vi "HFRR ADV v01.vi"() -> ()   [LabVIEW 2025] (continued)
  # "Choose which temperature sensor you are calibrating. Both use the same two-\npoint procedure: 0 °C (ice-point) and 60 °C (high-point)."
  # "Step 1 — Reference Instrument Setup"
  # "Connect a calibrated reference to the DUT port. This calibration performs two sets: one at 0 °C and one at 60 °C."
  # "Set A\n0 °C\nIce-point calibration"
  # "Set B\n60 °C\nHigh-point calibration"
  # "Allow the temperature bath to stabilise for at least 2 minutes at each set-point before recording the reading."
  # "Step 2 — Set A:  0 °C Calibration"
  # "Connect the  0 °C reference connector. Wait for the temperature to stabilise. Once stable, and click Record Point."
  # "Step 3 — Set B:  60 °C Calibration"
  # "Connect the  60 °C reference connector. Wait for the temperature to stabilise. Once stable, and click Record Point."
  # "Sample Temperature Calibration Complete"
  # "Sample Temperature Calibration PASSED\nMax deviation 0.200 °C — within ±0.5 °C tolerance. Two-point correction applied (0 °C & 60 °C)."
  # "Sample  Temperature Calibration Failed\nmeasured Sample Temperature differs from the factory calibration value"
  # "Step 1 — Reference Instrument Setup"
  # "Connect a calibrated reference to the DUT port. This calibration performs two sets: one at 0 °C and one at 60 °C."
  # "Set A\n0 °C\nIce-point calibration"
  # "Set B\n60 °C\nHigh-point calibration"
  # "Allow the temperature bath to stabilise for at least 2 minutes at each set-point before recording the reading."
  # "Step 2 — Set A:  0 °C Calibration"
  # "Connect the  0 °C reference connector. Wait for the temperature to stabilise. Once stable, and click Record Point."
  # "Step 3 — Set B:  60 °C Calibration"
  # "Connect the  60 °C reference connector. Wait for the temperature to stabilise. Once stable, and click Record Point."
  # "Air Temperature Calibration Complete"
  # "Air Temperature Calibration PASSED\nMax deviation 0.200 °C — within ±0.5 °C tolerance. Two-point correction applied (0 °C & 60 °C)."
  # "Air  Temperature Calibration Failed\nmeasured Sample Temperature differs from the factory calibration value"
  # "PID SAVE PARAMETERS"
  # "STROKE CALIBRATION"
  # "FF CALIBRATION"
  # "ABOUT SCREEN SAVE PARAMETERS"
  # "© 2023"
  # "System Control Commands\nS;1 - Starts the full automation cycle (Runs Priming-humidify till 70RH sequence first, then switches to Maintenance).\nS;0 - Stops the system immediately and enters Standby mode (Safe State: All actuators OFF).\nM;1 - Skips the priming sequence and jumps directly to Maintenance mode (PID control).\nR;1 - Resets the logic state machine and clears all errors, returning to Standby.\nService Mode (Manual Control)\nX;1 - Enters Manual Service Mode. This disables all automatic logic, sensor safety checks, and timers.\nX;0 - Exits Manual Service Mode and returns to Standby (Safe State).\nActuator Commands (Only work after sending X;1)\nP;[0-255] - Sets the Pump PWM. Note that this is Active Low (0 = Max Flow, 255 = Pump OFF).\nF;I;[0-255] - Sets the Intake Fan speed (0 = OFF, 255 = Max Speed).\nF;O;[0-255] - Sets the Exhaust Fan speed (0 = OFF, 255 = Max Speed).\nD;1 - Turns the Dehumidifier Relay ON.\nD;0 - Turns the Dehumidifier Relay OFF."
  # "%RH"
types:
  T1 = enum32{"Home", "Dashboard", "Imaging", "Report", "Analysis", "About", "Test Setup", "Advance", "Calibration"}
  T2 = typedef "imagedata.ctl" = cluster{"image type":i32, "image depth":i32, "image":u8[], "mask":u8[], "colors":u32[], "Rectangle":cluster{"left":i16, "top":i16, "right":i16, "bottom":i16}}
  T3 = enum32{"HOME", "Test Setup", "Acquire", "Compare Files", "Print Report", "About", "Advance", "Mooha"}
  T4 = enum32{"HOME", "Test Setup", "Acquire", "Adv Scar", "Adv Scar Report", "Compare Files", "Calibration", "About", "Advance", "Mooha"}
  T5 = enum16{"ASTM D6079", "ISO 12156", "CEC F-096-A-06", "Custom"}
  T6 = enum32{"Dashboard 1", "Dashboard 2", "Dashboard 3"}
  T7 = enum32{"COF", "Friction", "ECR", "Temperature", "Stroke"}
  T8 = enum32{"Coefficient Of Friction", "Air Temperature", "Humidity", "Stroke", "Sample Temperature", "Electrical Contact Resistance", "Frequency", "Air Temp vs Rh"}
  T9 = enum32{"Main", "Stroke", "Friction", "Temperature"}
  T10 = enum32{"Stroke Calibration", "Friction Force Calibration", "Temperature Calibration", "Default"}
  T11 = enum32{"Step 1", "Step 2", "Step 3", "Step 4", "Step 5", "Step 6", "Step 7", "Step 8", "Step 9"}
  T12 = enum32{"Test Progress", "Stroke Points Completed"}
  T13 = enum32{"Page 1", "Page 2", "Page 3", "Page 4", "Page 5", "Page 6"}
  T14 = enum32{"Main", "Step 1", "Step 2", "Step 3", "Step 4", "Air Step 1", "Air Step 2", "Air Step 3", "Air Step 4"}
  T15 = enum32{"Air Temperature", "Sample Temperature", "Default"}
  T16 = enum32{"COMMUNICATION", "CALIBRATION", "Temp Variables", "Camera", "WO 2472 (1)", "WO 2472 (2)", "WO 2472 (3)"}
  T17 = typedef "Auto Start enum.ctl" = enum16{"Init", "Humidity & Temperature On", "Reach point", "Maintain Stage", "Start Stage", "close", "Exit"}
  T18 = cluster{"Read Heave and Surge":string, "Bytes at Heave Port":dbl, "Heave and Surge COM Port:":refnum<visa-resource-name>, "Com Port 2":refnum<visa-resource-name>, "Residual Due":string, "Heave COM Status 2":bool, "Heave COM Status":bool, "Port 2":bool, "Sway PPR":dbl, "Surge PPR":dbl, "Heave PPR":dbl, "Sway Pitch":dbl, "Surge Pitch":dbl, "Heave Pitch":dbl, "Sway Pulses/mm":dbl, "Surge Pulses/mm":dbl, "Heave Pulses/mm":dbl, "inner loop":dbl, "Read Heave and Surge 2":string, "String 36":string, "Write S":bool, "WriteCC1":string[], "Heave COM Loop":i32, "LastCom":string, "EXIT":bool, "Error Heave":errorcluster}
  T19 = enum8{"Enabled", "Disabled", "Disabled and Grayed Out"}
  T20 = cluster{"Read Uno":string, "Bytes at Heave Port":dbl, "UNO COM Port:":refnum<visa-resource-name>, "UNO COM Port: 2":refnum<visa-resource-name>, "Residual Due":string, "UNO COM Status 2":bool, "UNO COM Status":bool, "Port 2":bool, "Sway PPR":dbl, "Surge PPR":dbl, "Heave PPR":dbl, "Sway Pitch":dbl, "Surge Pitch":dbl, "Heave Pitch":dbl, "Sway Pulses/mm":dbl, "Surge Pulses/mm":dbl, "Heave Pulses/mm":dbl, "inner loop":dbl, "Read Heave and Surge 2":string, "String 36":string, "Write S":bool, "WriteCC1":string[], "Heave COM Loop":i32, "LastCom":string, "EXIT":bool, "Error Heave":errorcluster}
  T21 = enum32{"HOME", "Test Setup", "Acquire", "Adv Scar", "Adv Scar Report", "Compare Files", "About", "Advance", "Mooha"}
  T22 = typedef "POST ANALYSIS ENUM.ctl" = enum16{"OPEN EXE", "INIT", "OPEN FILE", "FIT", "DRAW REC", "DRAW LINE", "PAN", "ZOOM IN", "ZOOM OUT", "SET ZOOM", "CLEAR ROI", "GET MEASUREMENTS", "RESIZE MODE", "STREAM START", "STREAM STOP", "SHOW UI", "MINIMIZE UI", "HIDE UI", "CKISE APP", "CLOSE CONNECTION", "SAVE IMAGE", "SET ROI COLOR", "READ", "TCP CHECK", "CLOSE"}
  T23 = typedef "CAMERA LIVE FEED ENUM.ctl" = enum16{"OPEN EXE", "INIT", "READ", "CAMERA CONNECT", "CAMERA START", "CAMERA STOP", "CAMERA GRAY", "CAMERA RGB", "CAMERA MINIMIZE", "CAMERA CLOSE", "CAMERA MODE LIST", "CAMERA MODE SET", "CAMERA RESTORE", "CAMERA SAVE", "CLOSE"}
  T24 = enum16{"Always On", "Always Off", "Off While Running"}
  T25 = enum32{"Home", "Dashboard", "Imaging", "Report", "Analysis", "About", "Test Setup", "Advance"}
  T26 = cluster{"File Name":string, "Test Method":string, "Operator":string, "Fuel Description":string, "Date and time":string}
  T27 = enum32{"Home", "Dashboard", "Imaging", "Report", "Analysis", "About", "Test Setup"}
  T28 = enum32{"HOME", "Test Setup", "Acquire", "Compare Files", "About", "Advance", "Mooha"}
  T29 = typedef "NI_ReportGenerationCore.lvlib/HTML Report Image Alignment.ctl" = enum16{"(default)", "LEFT", "RIGHT", "TOP", "TEXTTOP", "MIDDLE", "ABSMIDDLE", "BASELINE", "BOTTOM", "ABSBOTTOM"}
  T30 = cluster{"y":dbl, "LVDT STROKE DISPLAY":dbl, "y":dbl}
  T31 = enum16{"INIT", "READ", "MANUAL WRITE", "WRITE", "CLOSE", "ERROR INIT"}
diagram:
  w1 = FALSE
  w8 = 0.0 ("ch0_filt")
  w10 = -9999999.0 ("max_ch0")
  w11 = 9999999.0 ("min_ch0")
  w22 = FALSE ("Visible")
  w23 = T19."Enabled" ("Disabled")
  w26 = FALSE ("Visible")
  w25 = FALSE ("Humidity Off Command")
  w41 = "" ("USER ID")
  (unwired) T21."HOME" ("Main Tab")
  # "Temperature Continue Air Step 2"
  # "[CH1]    - FF\n[CH2]   - TEMPERATURE\n[CH3]    - Humidity\n[CH4]    - AIR TEMP\n[CH5]\\- Visa Uno\n[CH6] \\- Visa Due\n[CH7]  \\- file path\n[CH8]   - Displacement Gain\n[CHA]   - Stroke Gain\n[CHB]   - Stroke PID Gain\n[CHC]   -Language Selection\n[CHD]   -Power +\n[CHE]   -Power_\n[CHF]   -Heater\n[CHG]   -Humidity Wet\n[CHH]   -Humidity Dry\n[CHI]   -Integral Time \n[CHIJ   -Air intercept\n[CHI]   -Temp Intercept"
  n1 = local write "Cal Password"("" ("Cal Password")) -> ()
  n2 = property on="Auto Start Test" class="Bool (strict)"("Visible"=TRUE) -> ()  [unwired: 2 in, 2 out]
  n3 = property on="Friction Force Calibration Result Tab" class="TabCtl (strict)"("Visible"=FALSE) -> ()  [unwired: 2 in, 2 out]
  n4 = property on="FRICVALZ 2" class="Bool (strict)"("DisabledEnum"=w23) -> ()  [unwired: 2 in, 2 out]
  n5 = property on="FRICVALZ 4" class="Bool (strict)"("DisabledEnum"=w23) -> ()  [unwired: 2 in, 2 out]
  n6 = property on="FRICVALZ 3" class="Bool (strict)"("DisabledEnum"=w23) -> ()  [unwired: 2 in, 2 out]
  n7 = property on="About" class="Clust (strict)"("Visible"=FALSE) -> ()  [unwired: 2 in, 2 out]
  n8 = property on="Wrong Password" class="Str"("Visible"=w22) -> ()  [unwired: 2 in, 2 out]
  n9 = property on="Calibration 2" class="TabCtl (strict)"("Visible"=w22) -> ()  [unwired: 2 in, 2 out]
  n10 = local write "Temperature Selection"(T15."Default" ("Temperature Selection")) -> ()
  n11 = local write "Calibration Selection"(T10."Default" ("Calibration Selection")) -> ()
  n12 = flat-sequence {
    tunnel: [w77] -> w7
    tunnel: [w122] -> w33
    tunnel: w7 -> [w117]
    tunnel: [w123] -> w35
    tunnel: w33 -> [w123]
    tunnel: w35 -> [w183]
    tunnel: [w183] -> w34
    tunnel: w34 -> [w214]
    tunnel: [w214] -> w44
    tunnel: w44 -> [w221]
    tunnel: [w227] -> w32
    tunnel: [w215] -> w31
    tunnel: [w269] -> w6
    tunnel: [w268] -> _
    tunnel: w32 -> [w268]
    tunnel: w31 -> [w269]
    frame #0 {
      n13 = call "CLOSE CONNECTION.vi"("error in (no error)"="error in (no error) 2") -> ("error out"=w82:errorcluster)  [unwired: 10 in]
      n14 = call <vilib>:"Clear Errors.vi"("error in (no error)"=w82) -> ("error out"=w81:errorcluster)  [unwired: 5 in, 1 out]
      n15 = disable-structure shown="Enabled" {
        disable-tunnel: w81 -> [w109 _]
        disable-tunnel: [w108 _] -> w80
        frame Enabled {
          n16 = call <userlib>:"Fit VI window to Largest Dec.vi"("error in (no error)"=w109, "border spacing (2 px)"=1) -> ("error out"=w112:errorcluster, "dup VI Ref"=w116:refnum<vi>)  [unwired: 4 in]
          n17 = invoke on="Invoke Node" class="VI" method="FP.Run-Time Position.Maximized"(reference=w116, error in=w112) -> (error out=w113:errorcluster)  [unwired: 2 in, 3 out]
          n18 = call <vilib>:"Clear Errors.vi"("error in (no error)"=w113) -> ("error out"=w115:errorcluster)  [unwired: 5 in, 1 out]
          n19 = control-ref of="This VI"() -> (w107:refnum<vi>)
          n20 = invoke on="Invoke Node" class="VI" method="Default Vals.Reinit All"(reference=w107, error in=w115) -> (reference out=w111:refnum<vi>, error out=w110:errorcluster)  [unwired: 1 in, 1 out]
          n21 = Close Reference(reference=w111, error in (no error)=w110) -> (error out=w108:errorcluster)
        }
        frame Disabled {
        }
      }
      n22 = call "Stall Data Flow.vim"("value in"=w80, "milliseconds to wait"=u32 2000) -> ("value out"=w79:errorcluster)  [unwired: 1 out]
      n23 = call "Read Config.vi"("error in (no error)"=w79) -> ("error out"=w77:errorcluster, "STROKE PARAMETERS"=w88:dbl[], "ADC PARAMETERS"=w89:dbl[], "PID  PARAMETERS"=w90:dbl[], "CALIBRATION PARAMETERS"=w75:string[], "Stroke Calibration"=w87:string)  [unwired: 5 in]
      n24 = Index Array(array=w75) -> (element #1=w74:string, element #2=w73:string, element #3=w72:string, element #4=w71:string, element #5=w70:string, element #6=w68:string, element #7=w67:string, element #8=w66:string, element #9=w65:string, element #10=w64:string, element #11=w63:string, element #12=w62:string)  [unwired: 12 in]
      n25 = Index Array(array=w88) -> (element #1=w105:dbl, element #2=w106:dbl)  [unwired: 2 in]
      n26 = Index Array(array=w89) -> (element #1=w101:dbl, element #2=w102:dbl, element #3=w103:dbl, element #4=w104:dbl, element #5=w69:dbl)  [unwired: 5 in]
      n27 = Index Array(array=w90) -> (element #1=w92:dbl, element #2=w93:dbl, element #3=w94:dbl, element #4=w95:dbl, element #5=w96:dbl, element #6=w97:dbl, element #7=w98:dbl, element #8=w99:dbl, element #9=w100:dbl)  [unwired: 9 in]
      n28 = local write "STROKE FILTER"(w105) -> ()
      n29 = local write "Add up Stroke"(w106) -> ()
      n30 = local write "milliseconds to wait"(w92) -> ()
      n31 = local write "dt"(w93) -> ()
      n32 = local write "kp"(w94) -> ()
      n33 = local write "ki"(w95) -> ()
      n34 = local write "kd"(w96) -> ()
      n35 = local write "max_step_change"(w97) -> ()
      n36 = local write "max_amplitude"(w98) -> ()
      n37 = local write "min_amplitude"(w99) -> ()
      n38 = local write "startup_cmd"(w100) -> ()
      n39 = local write "VREF"(w101) -> ()
      n40 = local write "ADC_Resolution"(w102) -> ()
      n41 = local write "PIEZO_CAL_FACTOR"(w103) -> ()
      n42 = local write "NORMAL_FORCE"(w104) -> ()
      n43 = local write "Machine Serial Number"(w70) -> ()
      n44 = local write "STROKE CALIBRATION"(w74) -> ()
      n45 = local write "FRICTION CALIBRATION"(w73) -> ()
      n46 = local write "TEMPERATURE CALIBRATION"(w72) -> ()
      n47 = Fract/Exp String To Number(string=w71) -> (number=w76:dbl)  [unwired: 3 in, 1 out]
      n48 = local write "FF CAL EXCPTED VALUE"(w69) -> ()
      n49 = local write "version"(w68) -> ()
      n50 = local write "Version"(w67) -> ()
      n51 = local write "Workorder"(w66) -> ()
      n52 = local write "Runtime"(w65) -> ()
      n53 = local write "Firmware Version"(w64) -> ()
      n54 = local write "Operating System"(w63) -> ()
      n55 = local write "Instrument Serial"(w62) -> ()
      n56 = Spreadsheet String To Array(delimiter (Tab)=";", format string="", spreadsheet string=w87, array type (2D Dbl)=dbl[] []) -> (array=w91:dbl[])
      n57 = local write "Temperature diff"(w76) -> ()
      n58 = local write "calibration values"(w91) -> ()
    }
    frame #1 {
      n59 = property on="Auto Scar Check" class="Clust (strict)"("Visible"=TRUE) -> ()  [unwired: 2 in, 2 out]
      n60 = property on="Sign In" class="Bool (strict)"("DisabledEnum"=T19."Disabled" ("Disabled")) -> ()  [unwired: 2 in, 2 out]
      n61 = local write "sign in temp"(FALSE ("sign in temp")) -> ()
      n62 = call "dialog box.vi"("Status"="Before starting the test, verify that the microscope cable is connected.", "error in"=w117) -> ("error out"=w122:errorcluster)  [unwired: 8 in]
    }
    frame #2 {
      (unwired) TRUE ("Re-Initialise")
      # "kkkkk"
      # "C:\\Windows\\wndcm_pw_stdED hfrr.txt"
      # "C:\\LAB-IQ NXT"
      # "C:\\LAB-IQ NXT\\wndcm_pw_stdED hfrr.txt"
      # "password file"
      n63 = Current VI's Path() -> (path=w139:path)
      n64 = Strip Path(path=w139) -> (stripped path=w132:path)  [unwired: 1 out]
      n65 = local write "main tab sub"(enum32{"Page 1", "Page 2"}."Page 1" ("main tab sub")) -> ()
      n66 = local write "Main Tab Display"(T6."Dashboard 1" ("Main Tab Display")) -> ()
      n67 = local write "Main Tab"(T4."HOME" ("Main Tab")) -> ()
      n68 = Path To String(path=w132) -> (string=w134:string)
      n69 = Search/Split String(string=w134, search string/char (-)=".exe") -> (match + rest of string=w136:string)  [unwired: 1 in, 2 out]
      n70 = Match True/False String(2:".vi" ("false string"), 3:".exe" ("true string"), 4:w136) -> (0:w133:bool)  [unwired: 1 out]
      n71 = List Folder(path=path "C:/LAB-IQ" ("directory path"), pattern="*.txt") -> (filenames=w145:string[])  [unwired: 2 in, 3 out]
      n72 = case shown="True" w133 {
        tunnel: w132 -> [w154 w156]
        tunnel: [w154 w155] -> w130
        frame False {
        }
        frame True {
          n73 = Strip Path(path=w156) -> (stripped path=w155:path)  [unwired: 1 out]
        }
      }
      n74 = Search 1D Array(1D array=w145, element="wndcm_pw_stdED hfrr.txt") -> (index of element=w148:i32)  [unwired: 1 in]
      n75 = Equal?(x=w148, y=-1) -> (x = y?=w143:bool)
      n76 = Path To String(path=w130) -> (string=→"Gain path":string)
      n77 = case shown="True" w143 {
        frame False {
        }
        frame True {
          n78 = String To Byte Array(string="123\n") -> (unsigned byte array=w161:u8[])
          n79 = Array Size(array=w161) -> (size(s)=w160:i32)
          n80 = for {
            N: w160 -> [_]
            tunnel: w161 -> [w174]
            tunnel: [w171] -> w163 mode=indexing
            tunnel: w160 -> [w166]
            i -> [w164]
            n81 = Decrement(x=w166) -> (x-1=w167:i32)
            n82 = Index Array(array=w174, index=w164) -> (element=w173:u8)
            n83 = Equal?(x=w164, y=w167) -> (x = y?=w168:bool)
            n84 = Number To Decimal String(number=w173) -> (decimal integer string=w172:string)  [unwired: 1 in]
            n85 = Select(t="", s=w168, f="\r") -> (s? t:f=w165:string)
            n86 = Concatenate Strings(w172, w165) -> (w171:string)
          }
          n87 = local read "file path"() -> (w157:path)
          n88 = Concatenate Strings(w163) -> (w159:string)
          n89 = call <vilib>:"Write Characters To File.vi"("append to file? (new file:F)"=FALSE, "character string"=w159, "file path (dialog if empty)"=w157) -> ()  [unwired: 2 in, 1 out]
        }
      }
      n90 = local write "conststatus"(0.0 ("rpm value : 2")) -> ()
      n91 = local write "EVENT LOG"("") -> ()
      n92 = local write "COUNT"(0 ("COUNT")) -> ()
      n93 = local write "clk"(0.0 ("clk")) -> ()
      n94 = local write "Flag"(0.0 ("Flag")) -> ()
      n95 = local write "Lan flag"(0.0 ("Lan flag")) -> ()
      n96 = local write "Com flag"(u32 0 ("Com flag")) -> ()
      n97 = local write "refresh flag"(FALSE ("refresh flag")) -> ()
      "file path" <- path "C:/LAB-IQ/wndcm_pw_stdED hfrr.txt" ("file path")
      "FF buffer" <- dbl[] [] ("FF buffer")
    }
    frame #3 {
      # "C:\\WinDucom\\calibrate WO 2391.dcf"
      n98 = String To Path(string="C:\\LAB-IQ\\Image Calibrate v01.dcf") -> (path=w178:path)
      n99 = String To Path(string="C:\\LAB-IQ\\calibrate WO 2472.dcf") -> (path=w182:path)
      n100 = Open/Create/Replace File "Open File"(file path (use dialog)=w182) -> (refnum out=w181:refnum<file>)  [unwired: 5 in, 2 out]
      n101 = Open/Create/Replace File ("Open File")(file path (use dialog)=w178) -> (refnum out=w177:refnum<file>)  [unwired: 5 in, 2 out]
      n102 = for {
        N: 4 -> [_]
        tunnel: w177 -> [w189]
        i -> [w185]
        n103 = Read from Text File ("Read File")(file (use dialog)=w189) -> (text=w190:string)  [unwired: 3 in, 3 out]
        n104 = String Subset(string=w190, offset (0)=6, length (rest)=10 ("length (rest)")) -> (substring=w186:string)
        n105 = Fract/Exp String To Number(string=w186) -> (number=w184:dbl)  [unwired: 3 in, 1 out]
        n106 = case shown="3" w185 {
          tunnel: w184 -> [w191 w192 _ w193 _]
          frame 0 {
            n107 = local write "5x Gain"(w191) -> ()
          }
          frame 1 {
            n108 = local write "10x Gain"(w192) -> ()
          }
          frame 2 {
          }
          frame 3 {
            n109 = local write "100x gain"(w193) -> ()
          }
          frame 4, Default {
          }
        }
      }
      n110 = for {
        N: 24 -> [_]
        tunnel: w181 -> [w202]
        i -> [w196]
        (unwired) TRUE ("line mode (F)")
        n111 = Read from Text File "Read File"(file (use dialog)=w202) -> (text=w201:string)  [unwired: 3 in, 3 out]
        n112 = Match Pattern(string=w201, regular expression="]") -> (after substring=w199:string)  [unwired: 1 in, 3 out]
        n113 = String Subset(string=w201, offset (0)=5, length (rest)=10 ("length (rest)")) -> (substring=w194:string)
        n114 = Fract/Exp String To Number(string=w194) -> (number=w195:dbl)  [unwired: 3 in, 1 out]
        n115 = Match Pattern(string=w199, regular expression="-") -> (before substring=w197:string)  [unwired: 1 in, 3 out]
        n116 = case shown="18" w196 {
          tunnel: w195 -> [_ _ _ _ _ _ _ _ _ _ w209 _ _ _ _ _ _ _ _ _ _ _ _ _ _]
          tunnel: w197 -> [_ _ _ _ w205 w206 w207 _ _ _ _ _ _ _ _ _ _ _ _ _ w210 _ w211 w212 _]
          frame 0 {
          }
          frame 1 {
          }
          frame 2 {
          }
          frame 3 {
          }
          frame 4 {
            n117 = local write "Com Port 1"(w205) -> ()
          }
          frame 5 {
            n118 = local write "Com Port 2"(w206) -> ()
            n119 = local write "visa due"(w206) -> ()
          }
          frame 6 {
            n120 = String To Path(string=w207) -> (path=w208:path)
            n121 = local write "File Path"(w208) -> ()
          }
          frame 7 {
          }
          frame 8 {
          }
          frame 9 {
          }
          frame 10 {
            n122 = local write "Language Selection"(w209) -> ()
          }
          frame 11 {
          }
          frame 12 {
          }
          frame 13 {
          }
          frame 14 {
          }
          frame 15 {
          }
          frame 16 {
          }
          frame 17 {
          }
          frame 18 {
          }
          frame 21 {
          }
          frame 22 {
            n123 = local write "Com Port 3"(w210) -> ()
          }
          frame 23 {
          }
          frame 19 {
            n124 = local write "C3 :"(w211) -> ()
          }
          frame 20 {
            n125 = local write "Camera Port :"(w212) -> ()
          }
          frame 24, Default {
          }
        }
      }
    }
    frame #4 {
      n126 = Wait (ms)(milliseconds to wait=u32 1000) -> ()  [unwired: 1 out]
    }
    frame #5 {
      w230 = u32 2000 ("milliseconds to wait")
      w257 = u32 2000 ("milliseconds to wait")
      n127 = call "CAMERA LIVE FEED FGV.vi"("Enum - Menu"=CAMERA_LIVE_FEED_ENUM."OPEN EXE", "error in (no error)"=w221) -> ("error out"=w263:errorcluster)  [unwired: 8 in, 1 out]
      n128 = call "IMAGE ANALYSIS.vi"("Enum"=POST_ANALYSIS_ENUM."OPEN EXE", "error in"=w221) -> ("error out"=w218:errorcluster)  [unwired: 8 in, 1 out]
      n129 = call "Stall Data Flow.vim"("value in"=w263, "milliseconds to wait"=w257) -> ("value out"=w261:errorcluster)  [unwired: 1 out]
      n130 = call "Stall Data Flow.vim"("value in"=w218, "milliseconds to wait"=u32 8000) -> ("value out"=w217:errorcluster)  [unwired: 1 out]
      n131 = call "CAMERA LIVE FEED FGV.vi"("Enum - Menu"=CAMERA_LIVE_FEED_ENUM."INIT", "error in (no error)"=w261) -> ("error out"=w259:errorcluster)  [unwired: 8 in, 1 out]
      n132 = call "IMAGE ANALYSIS.vi"("Enum"=POST_ANALYSIS_ENUM."INIT", "error in"=w217) -> ("error out"=w215:errorcluster)  [unwired: 8 in, 1 out]
      n133 = case shown="Error .." w259 {
        selector: w259 -> [w264 _]
        tunnel: [w264 _] -> w258
        frame No Error {
        }
        frame Error {
          n134 = One Button Dialog(message="Camera initialization error.\nPlease Restart the software") -> ()  [unwired: 1 in, 1 out]
        }
      }
      n135 = property on="Camera Port :" class="CmbBox"() -> ("Strings[]"=w255:string[], "Value"=w256:string)  [unwired: 2 in, 2 out]
      n136 = Search 1D Array(1D array=w255, element=w256) -> (index of element=w254:i32)  [unwired: 1 in]
      n137 = Type Cast(type=30, x=w254) -> (*(type *) &x=w252:i32)
      n138 = call "Stall Data Flow.vim"("value in"=w258, "milliseconds to wait"=w257) -> ("value out"=w234:errorcluster)  [unwired: 1 out]
      n139 = Add(x=w252, y=48) -> (x+y=w233:i32)
      n140 = call "CAMERA LIVE FEED FGV.vi"("Enum - Menu"=CAMERA_LIVE_FEED_ENUM."CAMERA CONNECT", "error in (no error)"=w234, "CAMERA PORT"=w233) -> ("error out"=w243:errorcluster)  [unwired: 7 in, 1 out]
      n141 = call "Stall Data Flow.vim"("value in"=w243, "milliseconds to wait"=u32 5000) -> ("value out"=w244:errorcluster)  [unwired: 1 out]
      n142 = call "CAMERA LIVE FEED FGV.vi"("Enum - Menu"=CAMERA_LIVE_FEED_ENUM."CAMERA MODE LIST", "error in (no error)"=w244) -> ("error out"=w246:errorcluster)  [unwired: 8 in, 1 out]
      n143 = call "Stall Data Flow.vim"("value in"=w246, "milliseconds to wait"=w230) -> ("value out"=w245:errorcluster)  [unwired: 1 out]
      n144 = call "CAMERA LIVE FEED FGV.vi"("Enum - Menu"=CAMERA_LIVE_FEED_ENUM."READ", "error in (no error)"=w245) -> ("error out"=w232:errorcluster, "data out"=→"Camera List":string)  [unwired: 8 in]
      n145 = Type Cast(type=30, x=0) -> (*(type *) &x=w226:i32)
      n146 = call "Stall Data Flow.vim"("value in"=w232, "milliseconds to wait"=w230) -> ("value out"=w231:errorcluster)  [unwired: 1 out]
      n147 = Add(x=w226, y=48) -> (x+y=w224:i32)
      n148 = call "CAMERA LIVE FEED FGV.vi"("Enum - Menu"=CAMERA_LIVE_FEED_ENUM."CAMERA MODE SET", "error in (no error)"=w231, "CAMERA MODE"=w224) -> ("error out"=w228:errorcluster)  [unwired: 7 in, 1 out]
      n149 = call "Stall Data Flow.vim"("value in"=w228, "milliseconds to wait"=u32 2000) -> ("value out"=w248:errorcluster)  [unwired: 1 out]
      n150 = call "CAMERA LIVE FEED FGV.vi"("Enum - Menu"=CAMERA_LIVE_FEED_ENUM."CAMERA START", "error in (no error)"=w248) -> ("error out"=w249:errorcluster)  [unwired: 8 in, 1 out]
      n151 = call "Stall Data Flow.vim"("value in"=w249, "milliseconds to wait"=u32 1000) -> ("value out"=w250:errorcluster)  [unwired: 1 out]
      n152 = call "CAMERA LIVE FEED FGV.vi"("Enum - Menu"=CAMERA_LIVE_FEED_ENUM."CAMERA MINIMIZE", "error in (no error)"=w250) -> ("error out"=w227:errorcluster)  [unwired: 8 in, 1 out]
    }
    frame #6 {
      n153 = case shown="No Error" w268 {
        frame No Error {
          n154 = property on="Auto Scar Check" class="Clust (strict)"("Visible"=FALSE) -> ()  [unwired: 2 in, 2 out]
        }
        frame Error {
        }
      }
      n155 = property on="Sign In" class="Bool (strict)"("DisabledEnum"=T19."Enabled" ("Disabled")) -> ()  [unwired: 2 in, 2 out]
      n156 = local write "sign in temp"(TRUE ("sign in temp")) -> ()
    }
  }
  n157 = local write "SCAR MEASURMENT"(enum32{"Auto Scar", "Manual Scar"}."Manual Scar" ("SCAR MEASURMENT")) -> ()
  n158 = property on="Service Left" class="Bool (strict)"("Visible"=w1) -> ()  [unwired: 2 in, 2 out]
  n159 = property on="Service Right" class="Bool (strict)"("Visible"=w1) -> ()  [unwired: 2 in, 2 out]
  n160 = property on="Service Bottom" class="Bool (strict)"("Visible"=w1) -> ()  [unwired: 2 in, 2 out]
  n161 = local write "Temperature Off Command"(w25) -> ()
  n162 = local write "Main Dashboard Buttons"(T1."Home" ("Main Dashboard Buttons")) -> ()
  n163 = property on="Tab Control 6" class="TabCtl (strict)"("Visible"=FALSE) -> ()  [unwired: 2 in, 2 out]
  n164 = local write "Humidity Off Command"(w25) -> ()
  n165 = local write "CAMERA ROI MIN TEMP"(w25) -> ()
  n166 = local write "TEST FILE NAM,E SAVED"(w25) -> ()
  n167 = local write "LIVE FEED MIN TEMP"(w25) -> ()
  n168 = local write "SCAR MEASURMENT"(enum32{"Auto Scar", "Manual Scar"}."Manual Scar" ("SCAR MEASURMENT")) -> ()
  n169 = local write "Auto stop temp"(w26) -> ()
  n170 = local write "main tab sub"(enum32{"Page 1", "Page 2"}."Page 1" ("main tab sub")) -> ()
  n171 = while {
    stop <- w283 stop-if-true
    n172 = local read "Ambient Temperature"() -> (w281:dbl)
    n173 = Wait (ms)(milliseconds to wait=u32 200) -> ()  [unwired: 1 out]
    n174 = local read "Sample Temperature 2"() -> (w280:dbl)
    n175 = local write "Sensor value"(w281) -> ()
    n176 = local write "Sensor value"(w281) -> ()
    n177 = local write "Sensor value"(w280) -> ()
    n178 = local write "Sensor value"(w280) -> ()
    n179 = local write "Temperature — Live (Set A: 0 °C)"(w281) -> ()
    n180 = local write "Temperature — Live (Set A: 60 °C)"(w281) -> ()
    n181 = local write "Temperature — Live (Set A: 60 °C)"(w280) -> ()
    n182 = local write "Temperature — Live (Set A: 0 °C)"(w280) -> ()
    n183 = case shown="True" "Save Button" {
      selector: "Save Button" -> [_ w353]
      frame False {
      }
      frame True {
        n184 = Not(x=w353) -> (.not. x?=w352:bool)
        n185 = local read "Temperature diff"() -> (w349:dbl)
        n186 = local read "Machine Serial Number"() -> (w338:string)
        n187 = local read "milliseconds to wait"() -> (w385:u32)
        n188 = local write "Save Button"(w352) -> ()
        n189 = local read "max_step_change"() -> (w390:dbl)
        n190 = local read "FF CAL EXCPTED VALUE"() -> (w336:dbl)
        n191 = local read "Operating System"() -> (w329:string)
        n192 = local read "Firmware Version"() -> (w330:string)
        n193 = local read "max_amplitude"() -> (w391:dbl)
        n194 = local read "min_amplitude"() -> (w392:dbl)
        n195 = local read "Instrument Serial"() -> (w328:string)
        n196 = local read "PIEZO_CAL_FACTOR"() -> (w396:dbl)
        n197 = local read "startup_cmd"() -> (w393:dbl)
        n198 = local read "NORMAL_FORCE"() -> (w397:dbl)
        n199 = local read "ADC_Resolution"() -> (w395:dbl)
        n200 = local read "Workorder"() -> (w332:string)
        n201 = local read "Runtime"() -> (w331:string)
        n202 = local read "Version"() -> (w333:string)
        n203 = local read "version"() -> (w334:string)
        n204 = local read "kp"() -> (w387:dbl)
        n205 = local read "kd"() -> (w389:dbl)
        n206 = local read "calibration values"() -> (w400:dbl[])
        n207 = local read "dt"() -> (w386:dbl)
        n208 = local read "ki"() -> (w388:dbl)
        n209 = local read "STROKE FILTER"() -> (w398:i32)
        n210 = local read "Add up Stroke"() -> (w399:dbl)
        n211 = Number To Fractional String(number=w349) -> (F-format string=w348:string)  [unwired: 3 in]
        n212 = local read "VREF"() -> (w394:dbl)
        n213 = Insert Into Array(array=dbl[] [], new element #1=w385, new element #2=w386, new element #3=w387, new element #4=w388, new element #5=w389, new element #6=w390, new element #7=w391, new element #8=w392, new element #9=w393) -> (w401:dbl[])  [unwired: 1 in]
        n214 = Insert Into Array(array=dbl[] [], new element #1=w394, new element #2=w395, new element #3=w396, new element #4=w397, new element #5=w336) -> (w402:dbl[])  [unwired: 1 in]
        n215 = Array To Spreadsheet String(delimiter (Tab)=";", array=w400, 3:"" ("format string")) -> (spreadsheet string=w404:string)
        n216 = Insert Into Array(array=dbl[] [], new element #1=w398, new element #2=w399) -> (w403:dbl[])  [unwired: 1 in]
        n217 = Insert Into Array(array=string[] [], new element #1="STROKE CALIBRATION", new element #2="FRICTION CALIBRATION", new element #3="TEMPERATURE CALIBRATION", new element #4=w348, new element #5=w338, new element #6=w334, new element #7=w333, new element #8=w332, new element #9=w331, new element #10=w330, new element #11=w329, new element #12=w328) -> (w350:string[])  [unwired: 1 in]
        n218 = call "Write Config.vi"("Stroke Calibration"=w404, "CALIBRATION PARAMETERS"=w350, "STROKE PARAMETERS"=w403, "ADC PARAMETERS"=w402, "PID  PARAMETERS"=w401) -> ("error out"=w383:errorcluster)  [unwired: 6 in]
        n219 = call "Stall Data Flow.vim"("value in"=w383, "milliseconds to wait"=u32 2000) -> ("value out"=w384:errorcluster)  [unwired: 1 out]
        n220 = call "Read Config.vi"("error in (no error)"=w384) -> ("STROKE PARAMETERS"=w381:dbl[], "ADC PARAMETERS"=w380:dbl[], "PID  PARAMETERS"=w379:dbl[], "CALIBRATION PARAMETERS"=w344:string[], "Stroke Calibration"=w382:string)  [unwired: 5 in, 1 out]
        n221 = Index Array(array=w344) -> (element #1=w341:string, element #2=w340:string, element #3=w339:string, element #4=w343:string, element #5=w337:string, element #6=w327:string, element #7=w326:string, element #8=w325:string, element #9=w324:string, element #10=w323:string, element #11=w322:string, element #12=w321:string)  [unwired: 12 in]
        n222 = Index Array(array=w379) -> (element #1=w377:dbl, element #2=w376:dbl, element #3=w375:dbl, element #4=w374:dbl, element #5=w373:dbl, element #6=w372:dbl, element #7=w371:dbl, element #8=w370:dbl, element #9=w369:dbl)  [unwired: 9 in]
        n223 = Index Array(array=w380) -> (element #1=w368:dbl, element #2=w367:dbl, element #3=w366:dbl, element #4=w365:dbl, element #5=w335:dbl)  [unwired: 5 in]
        n224 = Index Array(array=w381) -> (element #1=w364:dbl, element #2=w363:dbl)  [unwired: 3 in, 1 out]
        n225 = Spreadsheet String To Array(delimiter (Tab)=";", format string="", spreadsheet string=w382, array type (2D Dbl)=dbl[] []) -> (array=w378:dbl[])
        n226 = local write "STROKE FILTER"(w364) -> ()
        n227 = local write "Add up Stroke"(w363) -> ()
        n228 = local write "VREF"(w368) -> ()
        n229 = local write "ADC_Resolution"(w367) -> ()
        n230 = local write "PIEZO_CAL_FACTOR"(w366) -> ()
        n231 = local write "NORMAL_FORCE"(w365) -> ()
        n232 = local write "FF CAL EXCPTED VALUE"(w335) -> ()
        n233 = local write "STROKE CALIBRATION"(w341) -> ()
        n234 = local write "FRICTION CALIBRATION"(w340) -> ()
        n235 = local write "TEMPERATURE CALIBRATION"(w339) -> ()
        n236 = Fract/Exp String To Number(string=w343) -> (number=w342:dbl)  [unwired: 3 in, 1 out]
        n237 = local write "Machine Serial Number"(w337) -> ()
        n238 = local write "version"(w327) -> ()
        n239 = local write "Version"(w326) -> ()
        n240 = local write "Workorder"(w325) -> ()
        n241 = local write "Runtime"(w324) -> ()
        n242 = local write "Firmware Version"(w323) -> ()
        n243 = local write "Operating System"(w322) -> ()
        n244 = local write "Instrument Serial"(w321) -> ()
        n245 = local write "calibration values"(w378) -> ()
        n246 = local write "milliseconds to wait"(w377) -> ()
        n247 = local write "dt"(w376) -> ()
        n248 = local write "kp"(w375) -> ()
        n249 = local write "ki"(w374) -> ()
        n250 = local write "kd"(w373) -> ()
        n251 = local write "max_step_change"(w372) -> ()
        n252 = local write "max_amplitude"(w371) -> ()
        n253 = local write "min_amplitude"(w370) -> ()
        n254 = local write "startup_cmd"(w369) -> ()
        n255 = local write "Temperature diff"(w342) -> ()
      }
    }
    n256 = local read "USER ID"() -> (w278:string)
    n257 = local read "run test Calibration"() -> (w276:bool)
    n258 = disable-structure shown="Enabled" {
      disable-tunnel: [w290 w301] -> w277
      frame Disabled {
        n259 = local read "Point 1 - 0.2 mm"() -> (w300:bool)
        n260 = local read "Point 2 - 0.4 mm"() -> (w299:bool)
        n261 = local read "Point 3 - 0.6 mm"() -> (w298:bool)
        n262 = local read "Point 4 - 0.8 mm"() -> (w297:bool)
        n263 = local read "Point 5 - 1.0 mm"() -> (w296:bool)
        n264 = local read "Point 6 - 1.2 mm"() -> (w295:bool)
        n265 = And(x=w300, y=w299) -> (x .and. y?=w294:bool)
        n266 = And(x=w298, y=w297) -> (x .and. y?=w293:bool)
        n267 = And(x=w296, y=w295) -> (x .and. y?=w291:bool)
        n268 = And(x=w294, y=w293) -> (x .and. y?=w292:bool)
        n269 = And(x=w292, y=w291) -> (x .and. y?=w290:bool)
      }
      frame Enabled {
        n270 = local read "Point 5 - 1.0 mm"() -> (w301:bool)
      }
    }
    n271 = local read "START TEMP"() -> (w275:bool)
    n272 = local write "tested by 2"(w278) -> ()
    n273 = And(x=w275, y=w276) -> (x .and. y?=w274:bool)
    n274 = case shown="True" w274 {
      frame False {
        w302 = TRUE ("PAUSE")
        n275 = call "ELAPSED TIMER VI - Calibration.vi"("RESET"=w302, "PAUSE"=w302) -> ()  [unwired: 7 in, 3 out]
      }
      frame True {
        w305 = FALSE ("PAUSE")
        n276 = call "ELAPSED TIMER VI - Calibration.vi"("TARGET"=60.0, "RESET"=w305, "PAUSE"=w305) -> ("ELAPSED INDICATION"=w303:bool)  [unwired: 6 in, 2 out]
        n277 = case shown="False" w303 {
          frame False {
            n278 = local write "Friction Force Calibration Result Tab"(enum32{"Calibration Results", "Page 2"}."Calibration Results" ("Friction Force Calibration Result Tab")) -> ()
            n279 = property on="Friction Force Calibration Result Tab" class="TabCtl (strict)"("Visible"=FALSE) -> ()  [unwired: 2 in, 2 out]
          }
          frame True {
            n280 = stacked-sequence {
              frame #0 {
                n281 = local read "Friction"() -> (→"Friction cal":dbl)
                n282 = local write "run test Calibration"(FALSE ("run test Calibration")) -> ()
                n283 = local write "START TEMP"(FALSE ("START TEMP")) -> ()
              }
              frame #1 {
                n284 = Wait (ms)(milliseconds to wait=u32 1500) -> ()  [unwired: 1 out]
              }
              frame #2 {
                n285 = local write "Due Write"("VC;0") -> ()
              }
              frame #3 {
                n286 = Wait (ms)(milliseconds to wait=u32 1500) -> ()  [unwired: 1 out]
              }
              frame #4 {
                n287 = local write "Due Write"("VC;0") -> ()
              }
              frame #5 {
                n288 = property on="Friction Force Calibration Result Tab" class="TabCtl (strict)"("Visible"=TRUE) -> ()  [unwired: 2 in, 2 out]
                n289 = property on="Tab Control 6" class="TabCtl (strict)"("Visible"=FALSE) -> ()  [unwired: 2 in, 2 out]
              }
            }
          }
        }
      }
    }
    n290 = local read "Friction cal"() -> (w273:dbl)
    n291 = case shown="False" w277 {
      frame False {
        n292 = property on="Accept & Save" class="Bool (strict)"("DisabledEnum"=T19."Disabled" ("Disabled")) -> ()  [unwired: 2 in, 2 out]
        n293 = property on="Tab Control 5" class="TabCtl (strict)"("Value"=enum32{"OK", "NG"}."NG" ("Tab Control 5")) -> ()  [unwired: 2 in, 2 out]
      }
      frame True {
        n294 = property on="Accept & Save" class="Bool (strict)"("DisabledEnum"=T19."Enabled" ("Disabled")) -> ()  [unwired: 2 in, 2 out]
        n295 = property on="Tab Control 5" class="TabCtl (strict)"("Value"=enum32{"OK", "NG"}."OK" ("Tab Control 5")) -> ()  [unwired: 2 in, 2 out]
      }
    }
    n296 = Greater Or Equal?(x=w273, y="FF CAL EXCPTED VALUE") -> (x >= y?=w271:bool)
    n297 = case shown="False" w271 {
      selector: w271 -> [w284 w287]
      frame False {
        n298 = local write "FF PASS"(w284) -> ()
        n299 = local write "Friction Force result Tab"(enum32{"OK", "NG"}."NG" ("Friction Force result Tab")) -> ()
        n300 = property on="Accept & Save FF" class="Bool (strict)"("DisabledEnum"=T19."Disabled" ("Disabled")) -> ()  [unwired: 2 in, 2 out]
      }
      frame True {
        n301 = local write "Friction Force result Tab"(enum32{"OK", "NG"}."OK" ("Friction Force result Tab")) -> ()
        n302 = property on="Accept & Save FF" class="Bool (strict)"("DisabledEnum"=T19."Enabled" ("Disabled")) -> ()  [unwired: 2 in, 2 out]
        "FF PASS" <- w287
      }
    }
    n303 = local read "Quit"() -> (w283:bool)
  }
  n304 = local write "USERNAME"(w41) -> ()
  n305 = local write "Main Tab"(T4."HOME" ("Main Tab")) -> ()
  n306 = local write "USER ID"(w41) -> ()
  n307 = property on="Auto Scar Check  2" class="Clust (strict)"("Visible"=w26) -> (error out=w29:errorcluster)  [unwired: 2 in, 1 out]
  n308 = property on="Quit" class="Bool (strict)"("Value"=FALSE ("Quit")) -> (error out=w43:errorcluster)  [unwired: 2 in, 1 out]
  n309 = while {
    stop <- w405 stop-if-true
    n310 = event shown="[11] \"Info\": Value Change" {
      selector: _ -> [_ _ _ _ _ _ _ _ _ _ _ _ _ _ _ _ _ _ _ _ _ _ _ _ _ _ _ _ _ _ _ _ _ _ _ _ _ _ _ _ _ _ _ _ _ _ _ _ _ _ _ _ _ _ _ _ _]
      dyn-events: _ -> [_ _ _ _ _ _ _ _ _ _ _ _ _ _ _ _ _ _ _ _ _ _ _ _ _ _ _ _ _ _ _ _ _ _ _ _ _ _ _ _ _ _ _ _ _ _ _ _ _ _ _ _ _ _ _ _ _]
      timeout: 100 -> [_ _ _ _ _ _ _ _ _ _ _ _ _ _ _ _ _ _ _ _ _ _ _ _ _ _ _ _ _ _ _ _ _ _ _ _ _ _ _ _ _ _ _ _ _ _ _ _ _ _ _ _ _ _ _ _ _]
      tunnel: [FALSE FALSE FALSE _ FALSE _ _ _ _ _ _ _ _ _ _ _ _ _ _ _ _ _ _ _ _ _ _ _ _ _ _ _ _ _ _ _ _ _ _ _ _ _ _ _ _ _ _ _ _ _ _ _ _ _ _ _ TRUE] -> w405
      event Timeout {
        n311 = event-data() -> ()  [unwired: 1 in, 3 out]
        n312 = disable-structure shown="Disabled" {
          frame Disabled {
            n313 = local read "Auto Start Test"() -> (w419:bool)
            n314 = local read "RUN"() -> (w420:bool)
            n315 = Or(x=w420, y=w419) -> (x .or. y?=w418:bool)
            n316 = case shown="True" w418 {
              frame False {
                w421 = TRUE ("PAUSE")
                n317 = call "ELAPSED TIMER VI - abort test.vi"("RESET"=w421, "PAUSE"=w421) -> ()  [unwired: 7 in, 3 out]
              }
              frame True {
                n318 = local read "Stroke 2"() -> (w426:dbl)
                n319 = local read "FF 3"() -> (w428:dbl)
                n320 = Equal?(x=w426, y=0.95 ("Stroke 2")) -> (x = y?=w423:bool)
                n321 = Equal?(x=w428, y=0.0 ("FF 3")) -> (x = y?=w424:bool)
                n322 = Or(x=w424, y=w423) -> (x .or. y?=w422:bool)
                n323 = case shown="True" w422 {
                  selector: w422 -> [_ w433]
                  frame False {
                    w429 = TRUE ("PAUSE")
                    n324 = call "ELAPSED TIMER VI - abort test.vi"("RESET"=w429, "PAUSE"=w429) -> ()  [unwired: 7 in, 3 out]
                  }
                  frame True {
                    n325 = Not(x=w433) -> (.not. x?=w432:bool)
                    n326 = call "ELAPSED TIMER VI - abort test.vi"("TARGET"=60.0, "RESET"=w432, "PAUSE"=FALSE) -> ("ELAPSED INDICATION"=w430:bool)  [unwired: 6 in, 2 out]
                    n327 = case shown="True" w430 {
                      frame False {
                      }
                      frame True {
                        n328 = stacked-sequence {
                          frame #0 {
                            w435 = FALSE
                            n329 = local write "RUN"(w435) -> ()
                            n330 = local write "Auto Start Test"(w435) -> ()
                          }
                          frame #1 {
                            n331 = One Button Dialog(message="Test stopped due to a communication error. Reconnect the C1 and C2 cables.") -> ()  [unwired: 1 in, 1 out]
                          }
                        }
                      }
                    }
                  }
                }
              }
            }
          }
          frame Enabled {
          }
        }
        n332 = Get Date/Time In Seconds() -> (seconds since 1Jan1904=w416:timestamp)
        n333 = Format Into String(format string="%<%m/%d/%Y %I:%M:%S %p>T", w416) -> (resulting string=→"Time Stamp":string)  [unwired: 2 in, 1 out]
        n334 = local read "Service Password enable"() -> (w408:bool)
        n335 = local read "FILE"() -> (w413:string)
        n336 = call <vilib>:"Trim Whitespace.vi"("string"=w413) -> ("trimmed string"=w412:string)  [unwired: 1 in]
        n337 = String Length(string=w412) -> (length=w411:i32)
        n338 = Greater?(x=w411, y=1) -> (0:w409:bool)
        n339 = case shown="False" w409 {
          tunnel: w408 -> [w437 _]
          frame False {
            n340 = case shown="False" w437 {
              frame True {
                w438 = "Test Start In Service Mode" ("Tip Strip")
